vi "Test3.vi"() -> ()   [LabVIEW 2013]
panel:
  out "standard error 2":string
  out "standard output 2":string
  out "standard error":string
  out "standard output":string
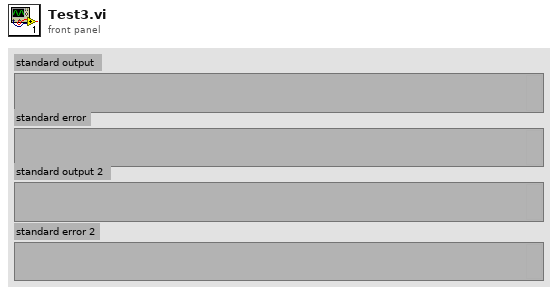
[diagram p1: front panel]
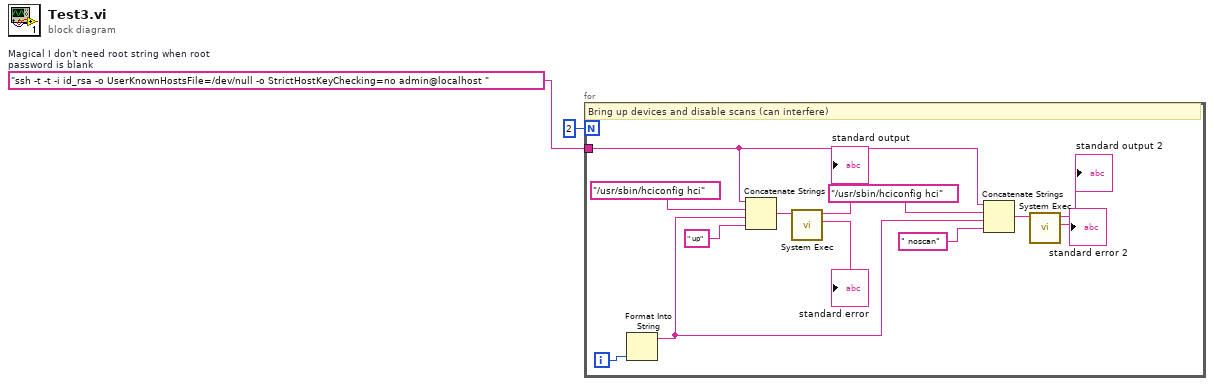
[diagram p0: block diagram]
diagram:
  w2 = "ssh -t -t -i id_rsa -o UserKnownHostsFile=/dev/null -o StrictHostKeyChecking=no admin@localhost "  # Magical I don't need root string when root password is blank
  n1 = for {
    N: 2 -> [_]
    tunnel: w2 -> [w7]
    i -> [w14]
    # "Bring up devices and disable scans (can interfere)"
    n2 = Format Into String(w14) -> (resulting string=w8:string)  [unwired: 3 in, 1 out]
    n3 = Concatenate Strings(w7, "/usr/sbin/hciconfig hci" ("command line"), w8, " up" ("string")) -> (w12:string)
    n4 = call <vilib>:"System Exec.vi"("command line"=w12) -> ("standard error"=→"standard error":string, "standard output"=→"standard output":string)  [unwired: 7 in, 2 out]
    n5 = Concatenate Strings(w7, "/usr/sbin/hciconfig hci" ("command line"), w8, " noscan" ("string")) -> (w11:string)
    n6 = call <vilib>:"System Exec.vi"("command line"=w11) -> ("standard error"=→"standard error 2":string, "standard output"=→"standard output 2":string)  [unwired: 7 in, 2 out]
  }
